vi "LV_alpha.vi"() -> ()   [LabVIEW 2021]
panel:
  out "x-y":dbl
  out "W22 Assignment 2 Q4 - Author: Ekin Yelken":cluster{dbl[], dbl[]}(graph)
  in  "Dial":i8(knob) scale=0.0..9.0
  in  "stop 2":bool
  out "7":bool
  out "5":bool
  out "3":bool
  out "6":bool
  out "4":bool
  out "2":bool
  out "1":bool
  out "W22 Assignment 2 Q2 - Author: Ekin Yelken":cluster{"Y":dbl[], "Y":dbl[]}[](graph)
  in  "stop":bool
  out "W22 Assignment 2 Q1 - Author: Ekin Yelken":cluster{"Knob":dbl, dbl}(graph)
  # "W22 Assignment 2 Q3 - Author: Ekin Yelken"
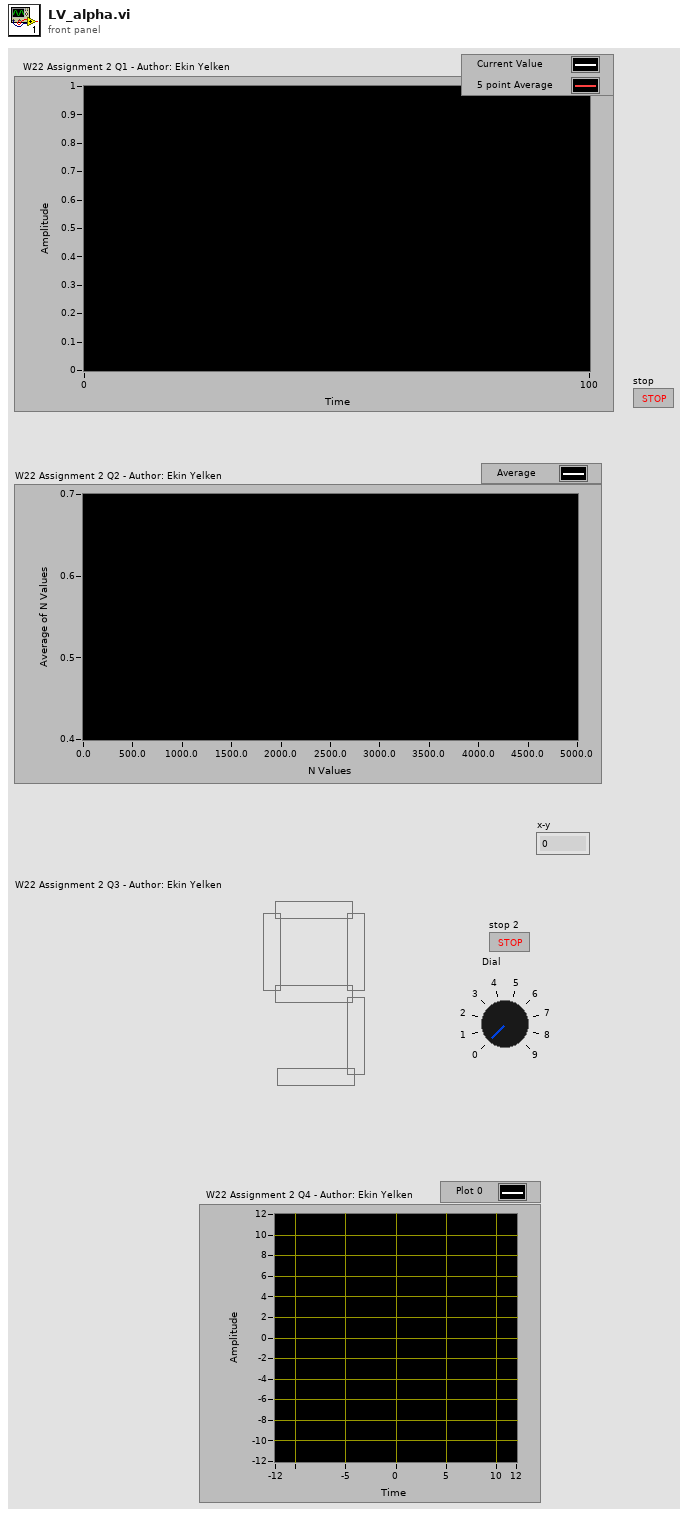
[diagram p1: front panel]
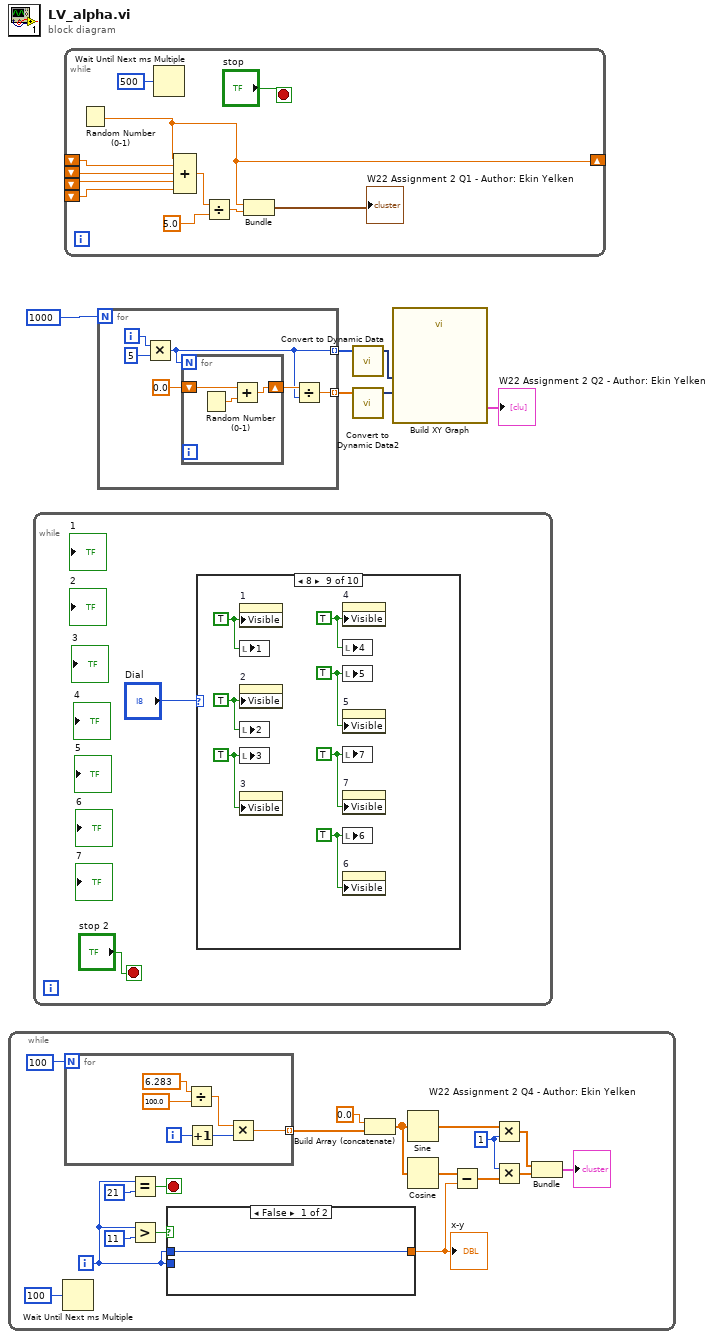
[diagram p0: block diagram]
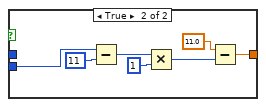
[diagram p2: hidden frame]
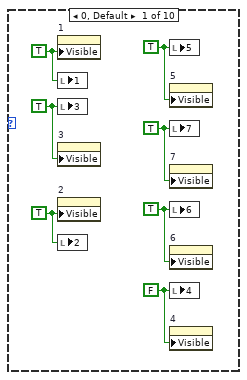
[diagram p3: hidden frame]
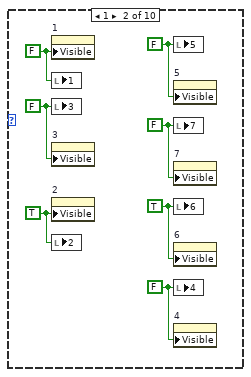
[diagram p4: hidden frame]
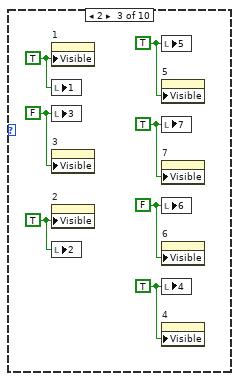
[diagram p5: hidden frame]
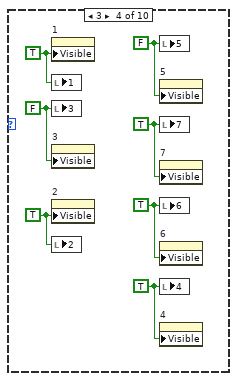
[diagram p6: hidden frame]
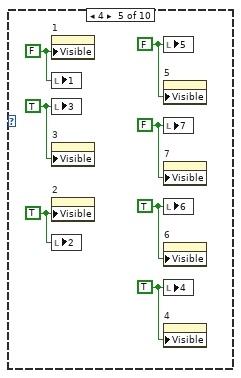
[diagram p7: hidden frame]
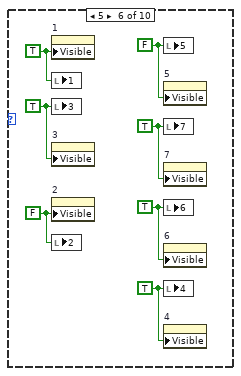
[diagram p8: hidden frame]
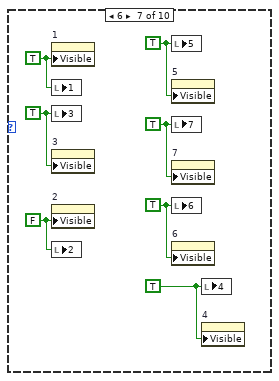
[diagram p9: hidden frame]
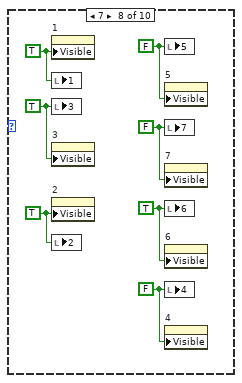
[diagram p10: hidden frame]
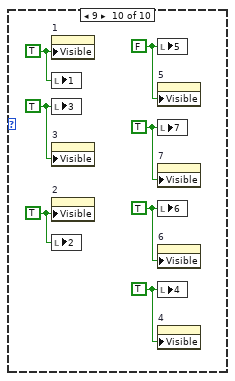
[diagram p11: hidden frame]
diagram:
  n1 = while {
    i -> [w8]
    stop <- w12 stop-if-true
    w22 = 1
    n2 = Wait Until Next ms Multiple(millisecond multiple=u32 100) -> ()  [unwired: 1 out]
    n3 = for {
      N: 100 -> [_]
      tunnel: [w34] -> w17 mode=indexing
      i -> [w37]
      n4 = Divide(x=6.283, y=100.0) -> (x/y=w36:dbl)
      n5 = Increment(x=w37) -> (x+1=w35:i32)
      n6 = Multiply(x=w36, y=w35) -> (x*y=w34:dbl)
    }
    n7 = Equal?(x=w8, y=21) -> (x = y?=w12:bool)
    n8 = Greater?(x=w8, y=11) -> (0:w10:bool)
    n9 = case shown="False" w10 {
      tunnel: w8 -> [w25 _]
      tunnel: [w25 w26] -> w7
      tunnel: w8 -> [_ w32]
      frame False {
      }
      frame True {
        n10 = Subtract(x=w32, y=11) -> (x-y=w30:i32)
        n11 = Multiply(x=w30, y=1) -> (x*y=w27:i32)
        n12 = Subtract(x=11.0, y=w27) -> (x-y=w26:dbl)
      }
    }
    "x-y" <- w7
    n13 = Build Array (concatenate)(0.0, w17) -> (w23:dbl[])
    n14 = Sine(x=w23) -> (sin(x)=w15:dbl[])
    n15 = Cosine(x=w23) -> (cos(x)=w13:dbl[])
    n16 = Subtract(x=w13, y=w7) -> (x-y=w14:dbl[])
    n17 = Multiply(x=w15, y=w22) -> (x*y=w18:dbl[])
    n18 = Multiply(x=w22, y=w14) -> (x*y=w19:dbl[])
    n19 = Bundle(w18, w19) -> (→"W22 Assignment 2 Q4 - Author: Ekin Yelken":cluster{dbl[], dbl[]})  [unwired: 1 in]
  }
  n20 = while {
    stop <- "stop 2" stop-if-true
    n21 = case shown="8" "Dial" {
      frame 0, Default {
        w45 = TRUE ("3")
        w43 = TRUE ("5")
        w41 = TRUE ("7")
        w42 = TRUE ("6")
        w44 = FALSE ("4")
        w46 = TRUE ("2")
        w47 = TRUE ("1")
        n22 = property on="1" class="Bool (strict)"("Visible"=w47) -> ()  [unwired: 2 in, 2 out]
        n23 = local write "1"(w47) -> ()
        n24 = local write "3"(w45) -> ()
        n25 = property on="3" class="Bool (strict)"("Visible"=w45) -> ()  [unwired: 2 in, 2 out]
        n26 = property on="2" class="Bool (strict)"("Visible"=w46) -> ()  [unwired: 2 in, 2 out]
        n27 = local write "2"(w46) -> ()
        n28 = local write "5"(w43) -> ()
        n29 = property on="5" class="Bool (strict)"("Visible"=w43) -> ()  [unwired: 2 in, 2 out]
        n30 = local write "7"(w41) -> ()
        n31 = property on="7" class="Bool (strict)"("Visible"=w41) -> ()  [unwired: 2 in, 2 out]
        n32 = local write "6"(w42) -> ()
        n33 = property on="6" class="Bool (strict)"("Visible"=w42) -> ()  [unwired: 2 in, 2 out]
        n34 = local write "4"(w44) -> ()
        n35 = property on="4" class="Bool (strict)"("Visible"=w44) -> ()  [unwired: 2 in, 2 out]
      }
      frame 1 {
        w54 = FALSE ("3")
        w53 = FALSE ("5")
        w52 = FALSE ("7")
        w51 = TRUE ("6")
        w50 = FALSE ("4")
        w49 = TRUE ("2")
        w48 = FALSE ("1")
        n36 = property on="1" class="Bool (strict)"("Visible"=w48) -> ()  [unwired: 2 in, 2 out]
        n37 = local write "1"(w48) -> ()
        n38 = local write "3"(w54) -> ()
        n39 = property on="3" class="Bool (strict)"("Visible"=w54) -> ()  [unwired: 2 in, 2 out]
        n40 = property on="2" class="Bool (strict)"("Visible"=w49) -> ()  [unwired: 2 in, 2 out]
        n41 = local write "2"(w49) -> ()
        n42 = local write "5"(w53) -> ()
        n43 = property on="5" class="Bool (strict)"("Visible"=w53) -> ()  [unwired: 2 in, 2 out]
        n44 = local write "7"(w52) -> ()
        n45 = property on="7" class="Bool (strict)"("Visible"=w52) -> ()  [unwired: 2 in, 2 out]
        n46 = local write "6"(w51) -> ()
        n47 = property on="6" class="Bool (strict)"("Visible"=w51) -> ()  [unwired: 2 in, 2 out]
        n48 = local write "4"(w50) -> ()
        n49 = property on="4" class="Bool (strict)"("Visible"=w50) -> ()  [unwired: 2 in, 2 out]
      }
      frame 2 {
        w59 = FALSE ("3")
        w57 = TRUE ("5")
        w55 = TRUE ("7")
        w56 = FALSE ("6")
        w58 = TRUE ("4")
        w60 = TRUE ("2")
        w61 = TRUE ("1")
        n50 = property on="1" class="Bool (strict)"("Visible"=w61) -> ()  [unwired: 2 in, 2 out]
        n51 = local write "1"(w61) -> ()
        n52 = local write "3"(w59) -> ()
        n53 = property on="3" class="Bool (strict)"("Visible"=w59) -> ()  [unwired: 2 in, 2 out]
        n54 = property on="2" class="Bool (strict)"("Visible"=w60) -> ()  [unwired: 2 in, 2 out]
        n55 = local write "2"(w60) -> ()
        n56 = local write "5"(w57) -> ()
        n57 = property on="5" class="Bool (strict)"("Visible"=w57) -> ()  [unwired: 2 in, 2 out]
        n58 = local write "7"(w55) -> ()
        n59 = property on="7" class="Bool (strict)"("Visible"=w55) -> ()  [unwired: 2 in, 2 out]
        n60 = local write "6"(w56) -> ()
        n61 = property on="6" class="Bool (strict)"("Visible"=w56) -> ()  [unwired: 2 in, 2 out]
        n62 = local write "4"(w58) -> ()
        n63 = property on="4" class="Bool (strict)"("Visible"=w58) -> ()  [unwired: 2 in, 2 out]
      }
      frame 3 {
        w67 = FALSE ("3")
        w66 = FALSE ("5")
        w65 = TRUE ("7")
        w64 = TRUE ("6")
        w63 = TRUE ("4")
        w62 = TRUE ("2")
        w68 = TRUE ("1")
        n64 = property on="1" class="Bool (strict)"("Visible"=w68) -> ()  [unwired: 2 in, 2 out]
        n65 = local write "1"(w68) -> ()
        n66 = local write "3"(w67) -> ()
        n67 = property on="3" class="Bool (strict)"("Visible"=w67) -> ()  [unwired: 2 in, 2 out]
        n68 = property on="2" class="Bool (strict)"("Visible"=w62) -> ()  [unwired: 2 in, 2 out]
        n69 = local write "2"(w62) -> ()
        n70 = local write "5"(w66) -> ()
        n71 = property on="5" class="Bool (strict)"("Visible"=w66) -> ()  [unwired: 2 in, 2 out]
        n72 = local write "7"(w65) -> ()
        n73 = property on="7" class="Bool (strict)"("Visible"=w65) -> ()  [unwired: 2 in, 2 out]
        n74 = local write "6"(w64) -> ()
        n75 = property on="6" class="Bool (strict)"("Visible"=w64) -> ()  [unwired: 2 in, 2 out]
        n76 = local write "4"(w63) -> ()
        n77 = property on="4" class="Bool (strict)"("Visible"=w63) -> ()  [unwired: 2 in, 2 out]
      }
      frame 4 {
        w72 = TRUE ("3")
        w71 = FALSE ("5")
        w69 = FALSE ("7")
        w70 = TRUE ("6")
        w73 = TRUE ("4")
        w74 = TRUE ("2")
        w75 = FALSE ("1")
        n78 = property on="1" class="Bool (strict)"("Visible"=w75) -> ()  [unwired: 2 in, 2 out]
        n79 = local write "1"(w75) -> ()
        n80 = local write "3"(w72) -> ()
        n81 = property on="3" class="Bool (strict)"("Visible"=w72) -> ()  [unwired: 2 in, 2 out]
        n82 = property on="2" class="Bool (strict)"("Visible"=w74) -> ()  [unwired: 2 in, 2 out]
        n83 = local write "2"(w74) -> ()
        n84 = local write "5"(w71) -> ()
        n85 = property on="5" class="Bool (strict)"("Visible"=w71) -> ()  [unwired: 2 in, 2 out]
        n86 = local write "7"(w69) -> ()
        n87 = property on="7" class="Bool (strict)"("Visible"=w69) -> ()  [unwired: 2 in, 2 out]
        n88 = local write "6"(w70) -> ()
        n89 = property on="6" class="Bool (strict)"("Visible"=w70) -> ()  [unwired: 2 in, 2 out]
        n90 = local write "4"(w73) -> ()
        n91 = property on="4" class="Bool (strict)"("Visible"=w73) -> ()  [unwired: 2 in, 2 out]
      }
      frame 5 {
        w79 = TRUE ("3")
        w78 = FALSE ("5")
        w76 = TRUE ("7")
        w77 = TRUE ("6")
        w80 = TRUE ("4")
        w81 = FALSE ("2")
        w82 = TRUE ("1")
        n92 = property on="1" class="Bool (strict)"("Visible"=w82) -> ()  [unwired: 2 in, 2 out]
        n93 = local write "1"(w82) -> ()
        n94 = local write "3"(w79) -> ()
        n95 = property on="3" class="Bool (strict)"("Visible"=w79) -> ()  [unwired: 2 in, 2 out]
        n96 = property on="2" class="Bool (strict)"("Visible"=w81) -> ()  [unwired: 2 in, 2 out]
        n97 = local write "2"(w81) -> ()
        n98 = local write "5"(w78) -> ()
        n99 = property on="5" class="Bool (strict)"("Visible"=w78) -> ()  [unwired: 2 in, 2 out]
        n100 = local write "7"(w76) -> ()
        n101 = property on="7" class="Bool (strict)"("Visible"=w76) -> ()  [unwired: 2 in, 2 out]
        n102 = local write "6"(w77) -> ()
        n103 = property on="6" class="Bool (strict)"("Visible"=w77) -> ()  [unwired: 2 in, 2 out]
        n104 = local write "4"(w80) -> ()
        n105 = property on="4" class="Bool (strict)"("Visible"=w80) -> ()  [unwired: 2 in, 2 out]
      }
      frame 6 {
        w86 = TRUE ("3")
        w85 = TRUE ("5")
        w83 = TRUE ("7")
        w84 = TRUE ("6")
        w87 = TRUE ("4")
        w88 = FALSE ("2")
        w89 = TRUE ("1")
        n106 = property on="1" class="Bool (strict)"("Visible"=w89) -> ()  [unwired: 2 in, 2 out]
        n107 = local write "1"(w89) -> ()
        n108 = local write "3"(w86) -> ()
        n109 = property on="3" class="Bool (strict)"("Visible"=w86) -> ()  [unwired: 2 in, 2 out]
        n110 = property on="2" class="Bool (strict)"("Visible"=w88) -> ()  [unwired: 2 in, 2 out]
        n111 = local write "2"(w88) -> ()
        n112 = local write "5"(w85) -> ()
        n113 = property on="5" class="Bool (strict)"("Visible"=w85) -> ()  [unwired: 2 in, 2 out]
        n114 = local write "7"(w83) -> ()
        n115 = property on="7" class="Bool (strict)"("Visible"=w83) -> ()  [unwired: 2 in, 2 out]
        n116 = local write "6"(w84) -> ()
        n117 = property on="6" class="Bool (strict)"("Visible"=w84) -> ()  [unwired: 2 in, 2 out]
        n118 = local write "4"(w87) -> ()
        n119 = property on="4" class="Bool (strict)"("Visible"=w87) -> ()  [unwired: 2 in, 2 out]
      }
      frame 7 {
        w95 = TRUE ("3")
        w92 = FALSE ("5")
        w90 = FALSE ("7")
        w91 = TRUE ("6")
        w93 = FALSE ("4")
        w94 = TRUE ("2")
        w96 = TRUE ("1")
        n120 = property on="1" class="Bool (strict)"("Visible"=w96) -> ()  [unwired: 2 in, 2 out]
        n121 = local write "1"(w96) -> ()
        n122 = local write "3"(w95) -> ()
        n123 = property on="3" class="Bool (strict)"("Visible"=w95) -> ()  [unwired: 2 in, 2 out]
        n124 = property on="2" class="Bool (strict)"("Visible"=w94) -> ()  [unwired: 2 in, 2 out]
        n125 = local write "2"(w94) -> ()
        n126 = local write "5"(w92) -> ()
        n127 = property on="5" class="Bool (strict)"("Visible"=w92) -> ()  [unwired: 2 in, 2 out]
        n128 = local write "7"(w90) -> ()
        n129 = property on="7" class="Bool (strict)"("Visible"=w90) -> ()  [unwired: 2 in, 2 out]
        n130 = local write "6"(w91) -> ()
        n131 = property on="6" class="Bool (strict)"("Visible"=w91) -> ()  [unwired: 2 in, 2 out]
        n132 = local write "4"(w93) -> ()
        n133 = property on="4" class="Bool (strict)"("Visible"=w93) -> ()  [unwired: 2 in, 2 out]
      }
      frame 8 {
        w102 = TRUE ("3")
        w101 = TRUE ("5")
        w99 = TRUE ("7")
        w98 = TRUE ("6")
        w97 = TRUE ("4")
        w100 = TRUE ("2")
        w103 = TRUE ("1")
        n134 = property on="1" class="Bool (strict)"("Visible"=w103) -> ()  [unwired: 2 in, 2 out]
        n135 = local write "1"(w103) -> ()
        n136 = property on="2" class="Bool (strict)"("Visible"=w100) -> ()  [unwired: 2 in, 2 out]
        n137 = local write "2"(w100) -> ()
        n138 = local write "3"(w102) -> ()
        n139 = property on="3" class="Bool (strict)"("Visible"=w102) -> ()  [unwired: 2 in, 2 out]
        n140 = property on="4" class="Bool (strict)"("Visible"=w97) -> ()  [unwired: 2 in, 2 out]
        n141 = local write "4"(w97) -> ()
        n142 = local write "5"(w101) -> ()
        n143 = property on="5" class="Bool (strict)"("Visible"=w101) -> ()  [unwired: 2 in, 2 out]
        n144 = local write "7"(w99) -> ()
        n145 = property on="7" class="Bool (strict)"("Visible"=w99) -> ()  [unwired: 2 in, 2 out]
        n146 = local write "6"(w98) -> ()
        n147 = property on="6" class="Bool (strict)"("Visible"=w98) -> ()  [unwired: 2 in, 2 out]
      }
      frame 9 {
        w108 = TRUE ("3")
        w106 = FALSE ("5")
        w104 = TRUE ("7")
        w105 = TRUE ("6")
        w107 = TRUE ("4")
        w109 = TRUE ("2")
        w110 = TRUE ("1")
        n148 = property on="1" class="Bool (strict)"("Visible"=w110) -> ()  [unwired: 2 in, 2 out]
        n149 = local write "1"(w110) -> ()
        n150 = local write "3"(w108) -> ()
        n151 = property on="3" class="Bool (strict)"("Visible"=w108) -> ()  [unwired: 2 in, 2 out]
        n152 = property on="2" class="Bool (strict)"("Visible"=w109) -> ()  [unwired: 2 in, 2 out]
        n153 = local write "2"(w109) -> ()
        n154 = local write "5"(w106) -> ()
        n155 = property on="5" class="Bool (strict)"("Visible"=w106) -> ()  [unwired: 2 in, 2 out]
        n156 = local write "7"(w104) -> ()
        n157 = property on="7" class="Bool (strict)"("Visible"=w104) -> ()  [unwired: 2 in, 2 out]
        n158 = local write "6"(w105) -> ()
        n159 = property on="6" class="Bool (strict)"("Visible"=w105) -> ()  [unwired: 2 in, 2 out]
        n160 = local write "4"(w107) -> ()
        n161 = property on="4" class="Bool (strict)"("Visible"=w107) -> ()  [unwired: 2 in, 2 out]
      }
    }
  }
  n162 = while {
    shift-right: [w113] -> _
    shift-left: _ -> [w117]
    shift-left: _ -> [w116]
    shift-left: _ -> [w115]
    shift-left: _ -> [w114]
    stop <- "stop" stop-if-true
    n163 = Random Number (0-1)() -> (number: 0 to 1=w113:dbl)
    n164 = Wait Until Next ms Multiple(millisecond multiple=u32 500) -> ()  [unwired: 1 out]
    n165 = Compound Arithmetic op=ADD(w113, w117, w116, w115, w114) -> (w120:dbl)
    n166 = Divide(x=w120, y=5.0) -> (x/y=w119:dbl)
    n167 = Bundle("number: 0 to 1"=w113, w119) -> (→"W22 Assignment 2 Q1 - Author: Ekin Yelken":cluster{"number: 0 to 1":dbl, dbl})  [unwired: 1 in]
  }
  n168 = for {
    N: 1000 -> [_]
    tunnel: [w123] -> w4 mode=indexing
    tunnel: [w122] -> w3 mode=indexing
    i -> [w127]
    n169 = Multiply(x=w127, y=5) -> (x*y=w122:i32)
    n170 = for {
      N: w122 -> [_]
      shift-right: [w129] -> w124
      shift-left: 0.0 -> [w128]
      n171 = Random Number (0-1)() -> (number: 0 to 1=w130:dbl)
      n172 = Add(x=w128, y=w130) -> (x+y=w129:dbl)
    }
    n173 = Divide(x=w124, y=w122) -> (x/y=w123:dbl)
  }
  n174 = call "Convert to Dynamic Data"("Array"=w3) -> ("Dynamic Data Type"=w2:dynamicdata)  [unwired: 3 in]
  n175 = call "Convert to Dynamic Data2"("Array"=w4) -> ("Dynamic Data Type"=w1:dynamicdata)  [unwired: 3 in]
  n176 = call "Build XY Graph"("Y Input"=w1, "X Input"=w2) -> ("XY Graph"=→"W22 Assignment 2 Q2 - Author: Ekin Yelken":cluster{"X":dbl[], "Y":dbl[]}[])  [unwired: 8 in, 1 out]
